vi "statistics.vi"() -> ()   [LabVIEW 2012]
uses:
  Trace controls.ctl
  probe_point.ctl
  <vilib>/Analysis/Matrix/Datatypes/RealMatrix.ctl
  pose_selector.ctl
  pose_source.ctl
  pose_relative_to.ctl
  <vilib>/Analysis/Matrix/Numeric/Conversions/Array To Matrix - RA.vi
  <vilib>/Analysis/Matrix/Numeric/Subtract/Subtract - RM,RM.vi
  <vilib>/Analysis/7linalg.llb/Real Eigenvalues and Vectors.vi
  <vilib>/Analysis/Matrix/Numeric/Complex/Complex To Cartesian - CM.vi
  <vilib>/Analysis/NI_AALPro.lvlib
  <vilib>/Analysis/4window.llb/Blackman-Harris Window (DBL).vi
  <vilib>/Analysis/4window.llb/windowTd.ctl
  <vilib>/Analysis/4window.llb/Window Properties by Name.vi
  <vilib>/gmath/NI_Gmath.lvlib
  <vilib>/Analysis/Matrix/NI_Matrix.lvlib
panel:
  out "max (overall)":dbl format="%#_3p"
  out "max":T1 format="%#_3p"
  in  "Pose B":T2[](array[typedef])
  in  "Pose A":T2[](array[typedef])
  in  "stop":bool
  out "sqrt(trace)":dbl format="%#_3p"
  out "sqrt(diag)":T1 format="%#_3p"
  in  "Decimate":i32=5
  out "1 - Correlation":T1 format="%#_3p"
  out "Correlation A x B":T1 format="%#_3p"
  in  "Group B":T5[](array[typedef])=[{"+ stim"=FALSE, "Relative"=FALSE, "Scale"=enum."1X", "Probe point"=enum."Output 0", "XYZ selector"={"Boolean"=TRUE, "Boolean 2"=TRUE, "Boolean 3"=TRUE}, "To tip"=FALSE}, {"+ stim"=FALSE, "Relative"=FALSE, "Scale"=enum."1X", "Probe point"=enum."Output 1", "XYZ selector"={"Boolean"=TRUE, "Boolean 2"=TRUE, "Boolean 3"=TRUE}, "To tip"=FALSE}, {"+ stim"=FALSE, "Relative"=FALSE, "Scale"=enum."1X", "Probe point"=enum."Position (tip)", "XYZ selector"={"Boolean"=FALSE, "Boolean 2"=FALSE, "Boolean 3"=FALSE}, "To tip"=FALSE}, {"+ stim"=FALSE, "Relative"=FALSE, "Scale"=enum."1X", "Probe point"=enum."Position (tip)", "XYZ selector"={"Boolean"=FALSE, "Boolean 2"=FALSE, "Boolean 3"=FALSE}, "To tip"=FALSE}]
  out "sqrt(eigenval)":T1 format="%#_3p"
  out "Eigenvectors":T1 format="%#.3g"
  out "Mean":T1 format="%#_3p"
  out "Covariance":T1 format="%#_3p"
  in  "Group A":T5[](array[typedef])=[{"+ stim"=FALSE, "Relative"=FALSE, "Scale"=enum."1X", "Probe point"=enum."Link residue 0", "XYZ selector"={"Boolean"=TRUE, "Boolean 2"=TRUE, "Boolean 3"=TRUE}, "To tip"=FALSE}, {"+ stim"=FALSE, "Relative"=FALSE, "Scale"=enum."1X", "Probe point"=enum."Link residue 1", "XYZ selector"={"Boolean"=TRUE, "Boolean 2"=TRUE, "Boolean 3"=TRUE}, "To tip"=FALSE}, {"+ stim"=FALSE, "Relative"=FALSE, "Scale"=enum."1X", "Probe point"=enum."Position (tip)", "XYZ selector"={"Boolean"=FALSE, "Boolean 2"=FALSE, "Boolean 3"=FALSE}, "To tip"=FALSE}, {"+ stim"=FALSE, "Relative"=FALSE, "Scale"=enum."1X", "Probe point"=enum."Position (tip)", "XYZ selector"={"Boolean"=FALSE, "Boolean 2"=FALSE, "Boolean 3"=FALSE}, "To tip"=FALSE}]
  # "Covariance"
  # "Correlation"
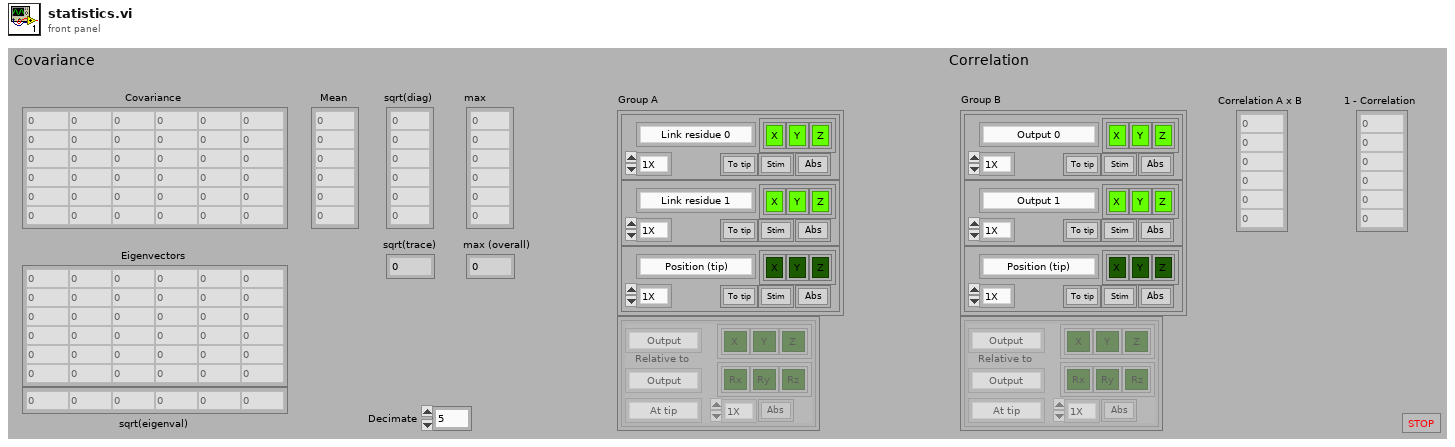
[diagram p1: front panel]
types:
  T1 = typedef "NI_Matrix.lvlib/RealMatrix.ctl" = dbl[][]
  T2 = typedef "pose_selector.ctl" = cluster{"Scale":enum16{"1X", "10X", "100X", "1KX", "10KX"}, "Source":T3, "XYZ selector":cluster{"Boolean":bool, "Boolean 2":bool, "Boolean 3":bool}, "RPY selector":cluster{"Boolean":bool, "Boolean 2":bool, "Boolean 3":bool}, "Relative to":T4, "Relative":bool, "Translate":enum16{"At tip", "At RCM", "At KC", "At origin"}}
  T3 = typedef "pose_source.ctl" = enum16{"Output", "Handle", "Handle KF", "Goal", "Absolute"}
  T4 = typedef "pose_relative_to.ctl" = enum16{"Output", "Handle", "Handle KF", "Goal", "Absolute", "Trace start"}
  T5 = typedef "Trace controls.ctl" = cluster{"+ stim":bool, "Relative":bool, "Scale":enum16{"1X", "10X", "100X", "1KX", "10KX"}, "Probe point":T6, "XYZ selector":cluster{"Boolean":bool, "Boolean 2":bool, "Boolean 3":bool}, "To tip":bool}
  T6 = typedef "probe_point.ctl" = enum16{"Position (tip)", "Position (RCM)", "Null pos (tip)", "Null pos (RCM)", "V limiter (tip)", "V Limiter (RCM)", "Goal (tip)", "Goal (RCM)", "Link pos 0", "Link pos 1", "KF link pos 0", "KF link pos 1", "Link rate 0", "Link rate 1", "Link residue 0", "Link residue 1", "Link goal 0", "Link goal 1", "Rate limit 0", "Rate limit 1", "Link error 0", "Link error 1", "Controller 0", "Controller 1", "Output 0", "Output 1", "Drive 0", "Drive 1", "Stimulus 0", "Stimulus 1", "Trace data 0", "Trace data 1", "Analog data 0", "Analog data 1", "Status flags", "Light 0", "Light 1", "Light 2", "Light 3", "Light 4", "Light 5", "Goal origin", "Goal rotation 0", "Goal rotation 1", "Goal rotation 2", "Output origin", "Output rotation 0", "Output rotation 1", "Output rotation 2", "Handle origin", "Handle rotation 0", "Handle rotation 1", "Handle rotation 2", "Handle position", "Handle velocity", "Handle acceleration", "Handle angles", "Handle angle rates", "Handle pos residue", "Handle angle residue", "Trace length"}
  T7 = typedef "NI_Matrix.lvlib/ComplexMatrix.ctl" = cdb[][]
  T8 = typedef "NI_AALPro.lvlib/windowTd.ctl" = u32
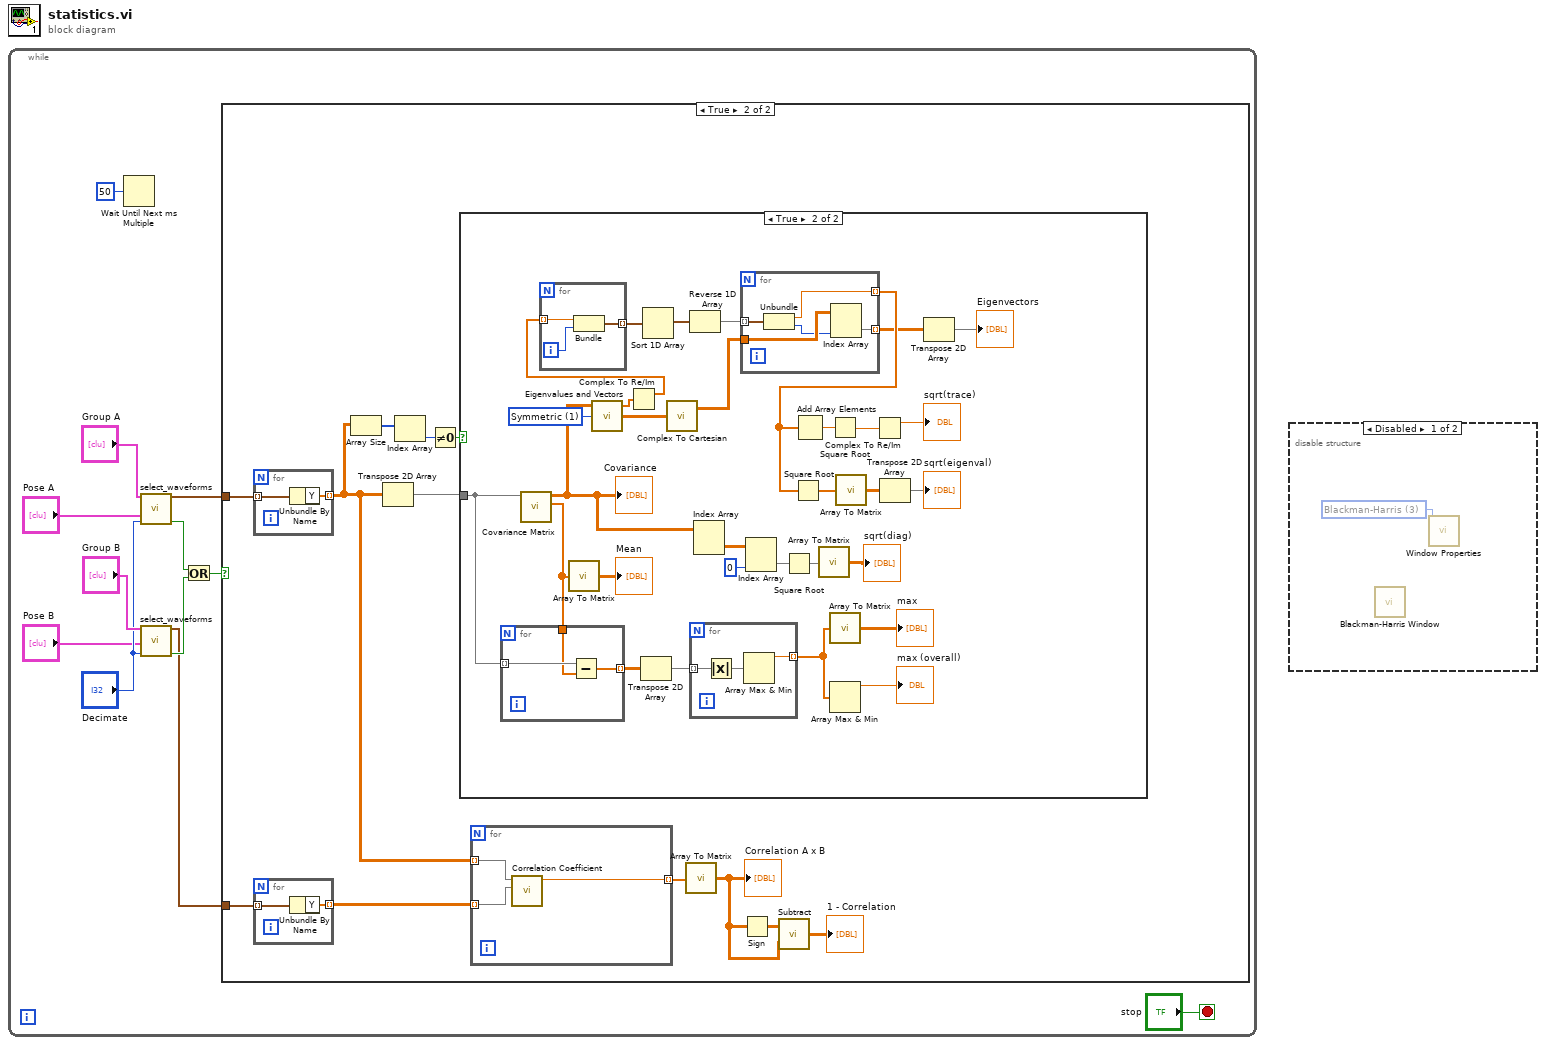
[diagram p0: block diagram]
diagram:
  n1 = while {
    stop <- "stop" stop-if-true
    n2 = Wait Until Next ms Multiple(millisecond multiple=u32 50) -> ()  [unwired: 1 out]
    n3 = call "select_waveforms.vi"("Trace controls"="Group A", "Pose selectors"="Pose A", "Decimate"="Decimate") -> ("Waveforms out"=w11:waveform(sgl)[], "New data"=w7:bool)  [unwired: 9 in, 2 out]
    n4 = call "select_waveforms.vi"("Trace controls"="Group B", "Pose selectors"="Pose B", "Decimate"="Decimate") -> ("Waveforms out"=w5:waveform(sgl)[], "New data"=w8:bool)  [unwired: 9 in, 2 out]
    n5 = Or(x=w7, y=w8) -> (x .or. y?=w6:bool)
    n6 = case shown="True" w6 {
      tunnel: w11 -> [_ w24]
      tunnel: w5 -> [_ w19]
      frame False {
      }
      frame True {
        n7 = for {
          tunnel: w24 -> [w76] mode=indexing
          tunnel: [w75] -> w18 mode=indexing
          n8 = Unbundle By Name(w76) -> ("Y"=w75:sgl[])
        }
        n9 = for {
          tunnel: w19 -> [w29] mode=indexing
          tunnel: [w28] -> w17 mode=indexing
          n10 = Unbundle By Name(w29) -> ("Y"=w28:sgl[])
        }
        n11 = Array Size(array=w18) -> (size(s)=w23:i32[])
        n12 = Transpose 2D Array(2D array=w18) -> (transposed array=w20:sgl[][])
        n13 = Index Array(array=w23) -> (element=w22:i32)  [unwired: 1 in]
        n14 = Not Equal To 0?(x=w22) -> (x != 0?=w21:bool)
        n15 = case shown="True" w21 {
          tunnel: w20 -> [_ w36]
          frame False {
          }
          frame True {
            w47 = 1 items=["General", "Symmetric"] ("matrix type")
            n16 = call <vilib>:"Covariance Matrix.vi"("X"=w36) -> ("mean vector"=w35:dbl[], "covariance matrix V"=w58:T1)  [unwired: 9 in]
            "Covariance" <- w58
            n17 = for {
              tunnel: w36 -> [w66] mode=indexing
              tunnel: w35 -> [w65]
              tunnel: [w64] -> w34 mode=indexing
              n18 = Subtract(x=w66, y=w65) -> (x-y=w64:dbl[])
            }
            n19 = call-poly <vilib>:"Array To Matrix.vi"("Real 1D Array"=w35) -> ("Real Matrix (Column Vector)"=→"Mean":T1)
            n20 = call-poly <vilib>:"Eigenvalues and Vectors.vi"("matrix type"=w47, "Input Matrix"=w58) -> ("Eigenvectors"=w40:T7, "Eigenvalues"=w46:cdb[])  [unwired: 1 in, 1 out]
            n21 = Complex To Re/Im(x + iy=w46) -> (x=w42:dbl[])  [unwired: 1 out]
            n22 = for {
              tunnel: w42 -> [w74] mode=indexing
              tunnel: [w72] -> w45 mode=indexing
              i -> [w73]
              n23 = Bundle(w74, w73) -> (w72:cluster{dbl, i32})  [unwired: 1 in]
            }
            n24 = Transpose 2D Array(2D array=w34) -> (transposed array=w33:dbl[][])
            n25 = Sort 1D Array(array=w45) -> (sorted array=w44:cluster{dbl, i32}[])
            n26 = call-poly <vilib>:"Complex To Cartesian.vi"("Complex Matrix R + Ii"=w40) -> ("Real Matrix R"=w39:T1)  [unwired: 1 out]
            n27 = Reverse 1D Array(array=w44) -> (reversed array=w43:cluster{dbl, i32}[])
            n28 = for {
              tunnel: w33 -> [w63] mode=indexing
              tunnel: [w61] -> w31 mode=indexing
              n29 = Absolute Value(x=w63) -> (abs(x)=w62:dbl[])
              n30 = Array Max & Min(array=w62) -> (max value=w61:dbl)  [unwired: 3 out]
            }
            n31 = Index Array(array=w58) -> (element=w57:T1)  [unwired: 2 in]
            n32 = for {
              tunnel: w43 -> [w71] mode=indexing
              tunnel: w39 -> [w70]
              tunnel: [w69] -> w38 mode=indexing
              tunnel: [w68] -> w41 mode=indexing
              n33 = Unbundle(w71) -> (w68:dbl, w67:i32)
              n34 = Index Array(array=w70, index (col)=w67) -> (element=w69:dbl[])  [unwired: 1 in]
            }
            n35 = Index Array(array=w57, index (col)=0 ("disabled index (col)")) -> (element=w50:dbl[])  [unwired: 1 in]
            n36 = Square Root ("Square Root.vi")(x=w50) -> (sqrt(x)=w55:dbl[])
            n37 = Square Root(x=w41) -> (sqrt(x)=w59:dbl[])
            n38 = Add Array Elements(numeric array=w41) -> (sum=w53:dbl)
            n39 = call-poly <vilib>:"Array To Matrix.vi"("Real 1D Array"=w55) -> ("Real Matrix (Column Vector)"=→"sqrt(diag)":T1)
            n40 = Square Root(x=w53) -> (sqrt(x)=w52:dbl)
            n41 = call-poly <vilib>:"Array To Matrix.vi"("Real 1D Array"=w31) -> ("Real Matrix (Column Vector)"=→"max":T1)
            n42 = Array Max & Min(array=w31) -> (max value=→"max (overall)":dbl)  [unwired: 3 out]
            n43 = call-poly <vilib>:"Array To Matrix.vi"("Real 1D Array"=w59) -> ("Real Matrix (Column Vector)"=w49:T1)
            n44 = Complex To Re/Im(x + iy=w52) -> (x=→"sqrt(trace)":dbl)  [unwired: 1 out]
            n45 = Transpose 2D Array(2D array=w49) -> (transposed array=→"sqrt(eigenval)":T1)
            n46 = Transpose 2D Array(2D array=w38) -> (transposed array=→"Eigenvectors":dbl[][])
          }
        }
        n47 = for {
          tunnel: w18 -> [w27] mode=indexing
          tunnel: w17 -> [w26] mode=indexing
          tunnel: [w25] -> w16 mode=indexing
          n48 = call <vilib>:"Correlation Coefficient.vi"("Y"=w26, "X"=w27) -> ("correlation coefficient r"=w25:dbl)  [unwired: 8 in, 1 out]
        }
        n49 = call-poly <vilib>:"Array To Matrix.vi"("Real 1D Array"=w16) -> ("Real Matrix (Column Vector)"=w14:T1)
        "Correlation A x B" <- w14
        n50 = Sign(1:w14) -> (0:w15:T1)
        n51 = call-poly <vilib>:"Subtract.vi"("Real Matrix B"=w14, "Real Matrix A"=w15) -> ("A - B"=→"1 - Correlation":T1)
      }
    }
  }
  n52 = disable-structure shown="Disabled" {
    frame Disabled {
      w77 = T8 3 items=["Rectangle"=0, "Hanning"=1, "Hamming"=2, "Blackman-Harris"=3, "Exact Blackman"=4, "Blackman"=5, "Flat Top"=6, "4 Term B-Harris "=7, "7 Term B-Harris"=8, "Low Sidelobe"=9, "Blackman Nuttall"=11, "Triangle"=30, "Bartlett-Hanning"=31, "Bohman"=32, "Parzen"=33, "Welch"=34, "Kaiser"=60, "Dolph-Chebyshev"=61, "Gaussian"=62] ("window")
      n53 = call-poly <vilib>:"Blackman-Harris Window.vi"() -> ()  [unwired: 1 in, 2 out]
      n54 = call-poly <vilib>:"Window Properties.vi"("window"=w77) -> ()  [unwired: 8 in, 3 out]
    }
    frame Enabled {
    }
  }
